vi "Setline_grouping_raw.vi"(8 "error in (no error)":errorcluster, 10 "Set_Val":i32, 11 "OneOfTemplate in":refnum<class "nidaqmx_grpc_CreateDOChanRequest_line_grouping_enum.lvclass">) -> (0 "error out":errorcluster, 3 "OneOfTemplate out":refnum<class "nidaqmx_grpc_CreateDOChanRequest_line_grouping_enum.lvclass">)   [LabVIEW 2021, in "NI_DAQmx_client.lvlib" / "nidaqmx_grpc_CreateDOChanRequest_line_grouping_enum.lvclass"]
uses:
  nidaqmx_grpc_CreateDOChanRequest_line_grouping_enum.lvclass
  nidaqmx_grpc_CreateDOChanRequest_line_grouping_enum.lvclass/nidaqmx_grpc_CreateDOChanRequest_line_grouping_enum.ctl
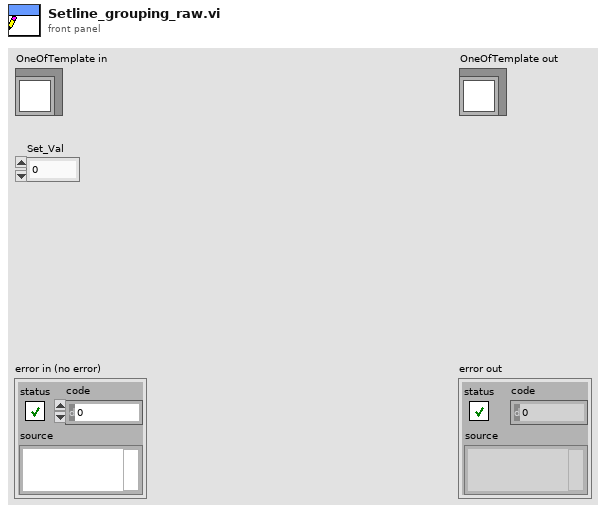
[diagram p1: front panel]
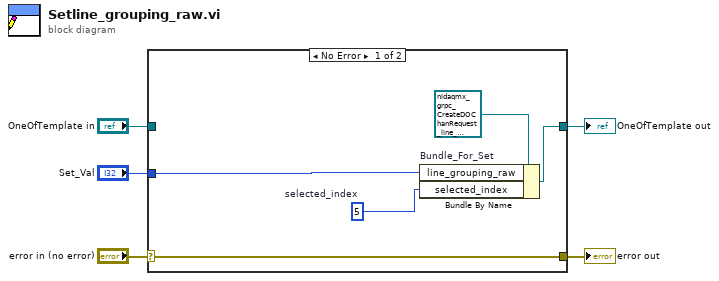
[diagram p0: block diagram]
diagram:
  n1 = case shown="No Error" "error in (no error)" {
    selector: "error in (no error)" -> [w10 w11]
    tunnel: [w10 w11] -> w4
    tunnel: [w9 w12] -> w2
    tunnel: "OneOfTemplate in" -> [_ w12]
    tunnel: "Set_Val" -> [w8 _]
    frame No Error {
      w7 = 5  # selected_index
      n2 = Bundle By Name "Bundle_For_Set"(cluster=refnum<class "nidaqmx_grpc_CreateDOChanRequest_line_grouping_enum.lvclass"> refnum ("OneOfTemplate in"), "line_grouping_raw"=w8, "selected_index"=w7) -> (w9:refnum<class "nidaqmx_grpc_CreateDOChanRequest_line_grouping_enum.lvclass">)
    }
    frame Error {
    }
  }
  "error out" <- w4
  "OneOfTemplate out" <- w2
